vi "PicoScope2000aIsReady.vi"(8 "error in (no error)":errorcluster, 11 "handle in":i16) -> (0 "error out":errorcluster, 3 "handle out":i16, 6 "ready":i16)   [LabVIEW 2010]
doc: "Calls IsReady"
uses:
  ps2000a.dll
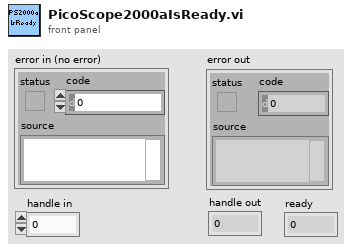
[diagram p1: front panel]
types:
  T1 = cluster{"status":bool, "code":u32, "source":string}
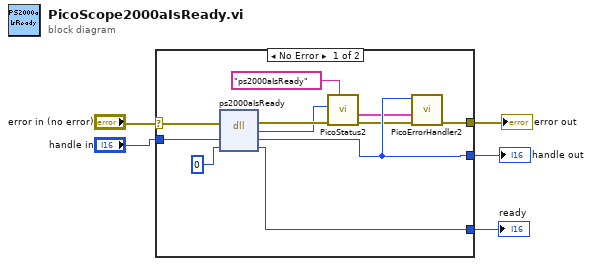
[diagram p0: block diagram]
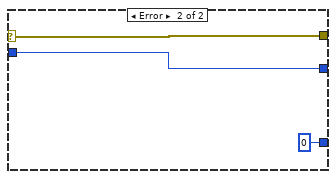
[diagram p2: hidden frame]
diagram:
  n1 = case shown="No Error" "error in (no error)" {
    selector: "error in (no error)" -> [w15 w18]
    tunnel: "handle in" -> [w16 w19]
    tunnel: [w12 w19] -> w5
    tunnel: [w7 w18] -> w4
    tunnel: [w8 i16 0 ("ready")] -> w3
    frame No Error {
      n2 = dll-call lib="ps2000a.dll" fn="ps2000aIsReady" ("ps3000.dll:_ps3000_open_unit@0")(error in=w15, "handle"=w16, "ready"=i16 0) -> (error out=w14:errorcluster, "PICO_STATUS"=w10:u32, "handle"=w12:i16, "ready"=w8:i16)  [unwired: 2 in, 1 out]
      n3 = call "PicoStatus2.vi"("PICO source"="ps2000aIsReady" ("source"), "Error in"=w14, "PICO STATUS"=w10) -> ("error out"=w9:errorcluster, "PICO_STATUS out"=w6:T1)  [unwired: 5 in]
      n4 = call "PicoErrorHandler2.vi"("error in (no error)"=w9, "PICO_STATUS in"=w6, "handle In"=w12) -> ("error out"=w7:errorcluster)  [unwired: 8 in]
    }
    frame Error {
    }
  }
  "error out" <- w4
  "handle out" <- w5
  "ready" <- w3
